vi "PM5000_VIF_Graficas.vi"(8 "error in":errorcluster, 11 "Network Path":string="172.22.26.202") -> (0 "error out":errorcluster, 2 "output cluster":T1, 3 "Network Path out":string="192.168.169.1")   [LabVIEW 2018]
doc: "Lee la tabla de memoria RealTime_VIF_Power del equipo PowerMonitor 5000, ademas filtra y ordena las variables de interez de la tabla de memoria.\n\nLee las siguientes variables de la tabla RealTime_VIF_Power:\n\n*V1_V2_Volts\n*V2_V3_Volts\n*V3_V1_Volts\n*I1_Amps\n*I2_Amps\n*I3_Amps\n*Frequency_Hz\n*Total_kW\n*Total_kVAR\n*Total_kVA\n*Total_True_PF\n*Total_Disp_PF"
uses:
  Controls/VIF_cluster.ctl
  <vilib>/ethernetip/ethernetip.llb/EthernetIP SLC500 Read Float.vi
  <vilib>/ethernetip/ethernetip.lvlib
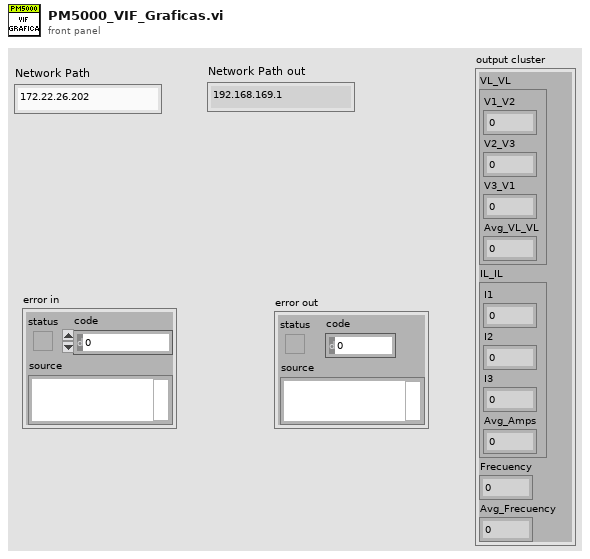
[diagram p1: front panel]
types:
  T1 = typedef "VIF_cluster.ctl" = cluster{"VL_VL":cluster{"V1_V2":sgl, "V2_V3":sgl, "V3_V1":sgl, "Avg_VL_VL":sgl}, "IL_IL":cluster{"I1":sgl, "I2":sgl, "I3":sgl, "Avg_Amps":sgl}, "Frecuency":sgl, "Avg_Frecuency":sgl}
  T2 = cluster{"I1":sgl, "I2":sgl, "I3":sgl, "Avg_Amps":sgl}
  T3 = cluster{"V1_V2":sgl, "V2_V3":sgl, "V3_V1":sgl, "Avg_VL_VL":sgl}
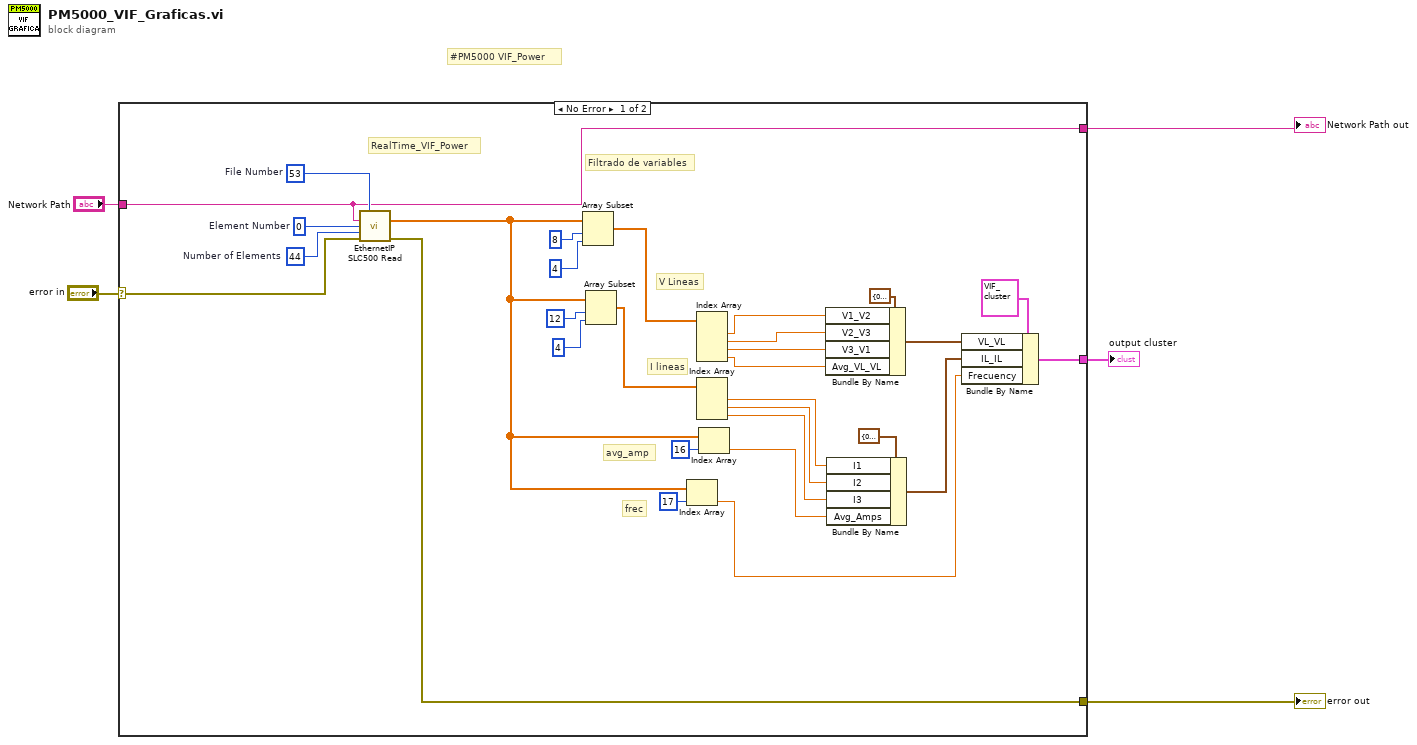
[diagram p0: block diagram]
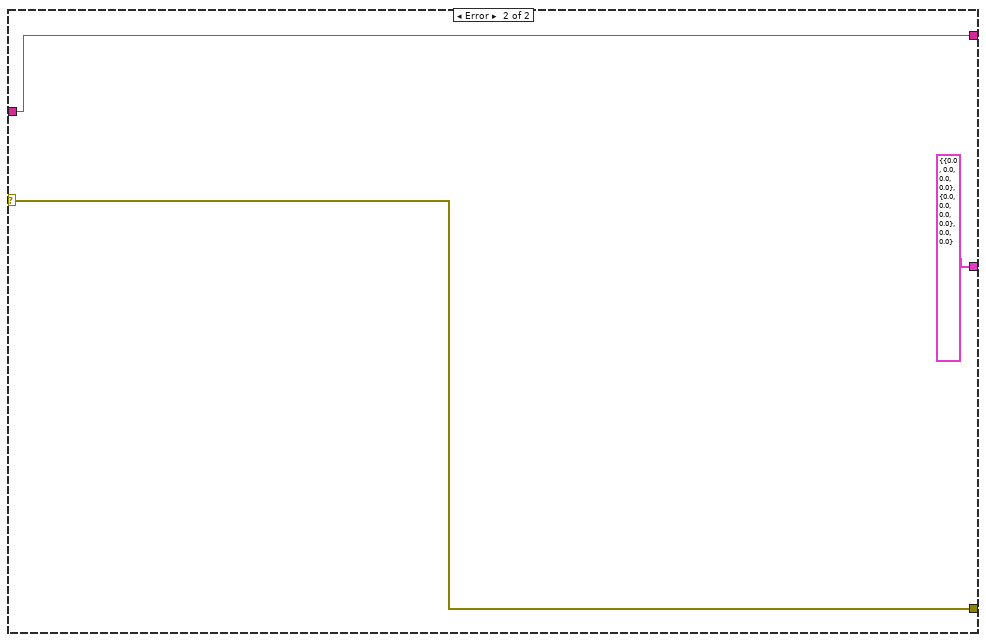
[diagram p2: hidden frame]
diagram:
  # "#PM5000 VIF_Power"
  n1 = case shown="No Error" "error in" {
    selector: "error in" -> [w27 w38]
    tunnel: [w32 w38] -> w5
    tunnel: [w24 w37] -> w3
    tunnel: "Network Path" -> [w24 w37]
    tunnel: [w9 T1 {"VL_VL"={"V1_V2"=0.0, "V2_V3"=0.0, "V3_V1"=0.0, "Avg_VL_VL"=0.0}, "IL_IL"={"I1"=0.0, "I2"=0.0, "I3"=0.0, "Avg_Amps"=0.0}, "Frecuency"=0.0, "Avg_Frecuency"=0.0} ("VIF_cluster")] -> w1
    frame No Error {
      w33 = u32 44  # Number of Elements
      w35 = u16 53  # File Number
      w34 = u16 0  # Element Number
      # "avg_amp"
      # "frec"
      # "I lineas"
      # "V Lineas"
      # "Filtrado de variables"
      # "RealTime_VIF_Power"
      n2 = call-poly <vilib>:"EthernetIP SLC500 Read.vi"("File Number"=w35, "Network Path"=w24, "Element Number"=w34, "Number of Elements"=w33, "error in"=w27) -> ("Data"=w8:sgl[], "error out"=w32:errorcluster)  [unwired: 8 in, 1 out]
      n3 = Array Subset(array=w8, index=8, length=4) -> (w26:sgl[])
      n4 = Array Subset(array=w8, index=12, length=4) -> (w25:sgl[])
      n5 = Index Array(array=w8, index=17) -> (element=w10:sgl)
      n6 = Index Array(array=w26) -> (element #1=w17:sgl, element #2=w16:sgl, element #3=w15:sgl, element #4=w14:sgl)  [unwired: 4 in]
      n7 = Index Array(array=w25) -> (element #1=w13:sgl, element #2=w12:sgl, element #3=w11:sgl)  [unwired: 3 in]
      n8 = Index Array(array=w8, index=16) -> (element=w6:sgl)
      n9 = Bundle By Name(cluster=T3 {"V1_V2"=0.0, "V2_V3"=0.0, "V3_V1"=0.0, "Avg_VL_VL"=0.0} ("VL_VL"), "V1_V2"=w17, "V2_V3"=w16, "V3_V1"=w15, "Avg_VL_VL"=w14) -> (w21:T3)
      n10 = Bundle By Name(cluster=T2 {"I1"=0.0, "I2"=0.0, "I3"=0.0, "Avg_Amps"=0.0} ("IL_IL"), "I1"=w13, "I2"=w12, "I3"=w11, "Avg_Amps"=w6) -> (w19:T2)
      n11 = Bundle By Name(cluster=T1 {"VL_VL"={"V1_V2"=0.0, "V2_V3"=0.0, "V3_V1"=0.0, "Avg_VL_VL"=0.0}, "IL_IL"={"I1"=0.0, "I2"=0.0, "I3"=0.0, "Avg_Amps"=0.0}, "Frecuency"=0.0, "Avg_Frecuency"=0.0} ("VIF_cluster"), "VL_VL"=w21, "IL_IL"=w19, "Frecuency"=w10) -> (w9:T1)
    }
    frame Error {
    }
  }
  "error out" <- w5
  "Network Path out" <- w3
  "output cluster" <- w1
